vi "Assert Floating Point wired to Floating Point Type.vi"   [LabVIEW 2017]
uses:
  b7307dac-1fbb-4763-be12-0bd798c1d309.vi
  455eed85-9c29-4121-af11-d9cb0bec3e29.vi
  b044ac8e-82c3-4b9a-a16b-66d0f1074277.vi
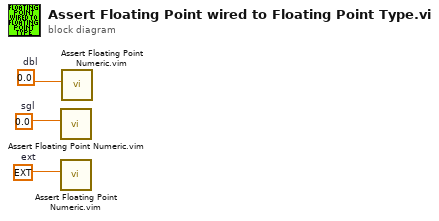
[diagram p0: block diagram]
diagram:
  w1 = ext 0.0  # ext
  w2 = sgl 0.0  # sgl
  w3 = 0.0  # dbl
  n1 = call "Assert Floating Point Numeric.vim"("Input"=w2) -> ()  [unwired: 10 in, 1 out]
  n2 = call "Assert Floating Point Numeric.vim"("Input"=w1) -> ()  [unwired: 10 in, 1 out]
  n3 = call "Assert Floating Point Numeric.vim"("Input"=w3) -> ()  [unwired: 10 in, 1 out]
